vi "addTaskMethod.vi"(8 "error in":errorcluster, 10 "stopMechanismType":T1, 11 "classPath":path) -> (0 "error out":errorcluster, 2 "taskViPath":path, 3 "classPath(dup)":path)   [LabVIEW 2023]
uses:
  stopMechanismType.ctl
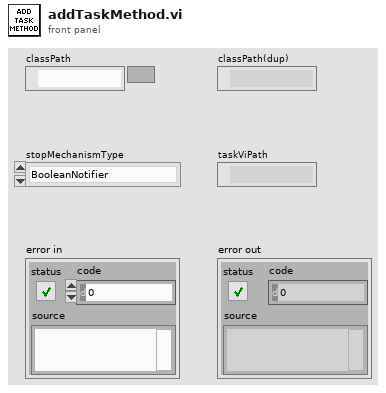
[diagram p1: front panel]
types:
  T1 = typedef "stopMechanismType.ctl" = enum16{"BooleanNotifier", "BooleanUE", "MsgUE", "MsgQueue"}
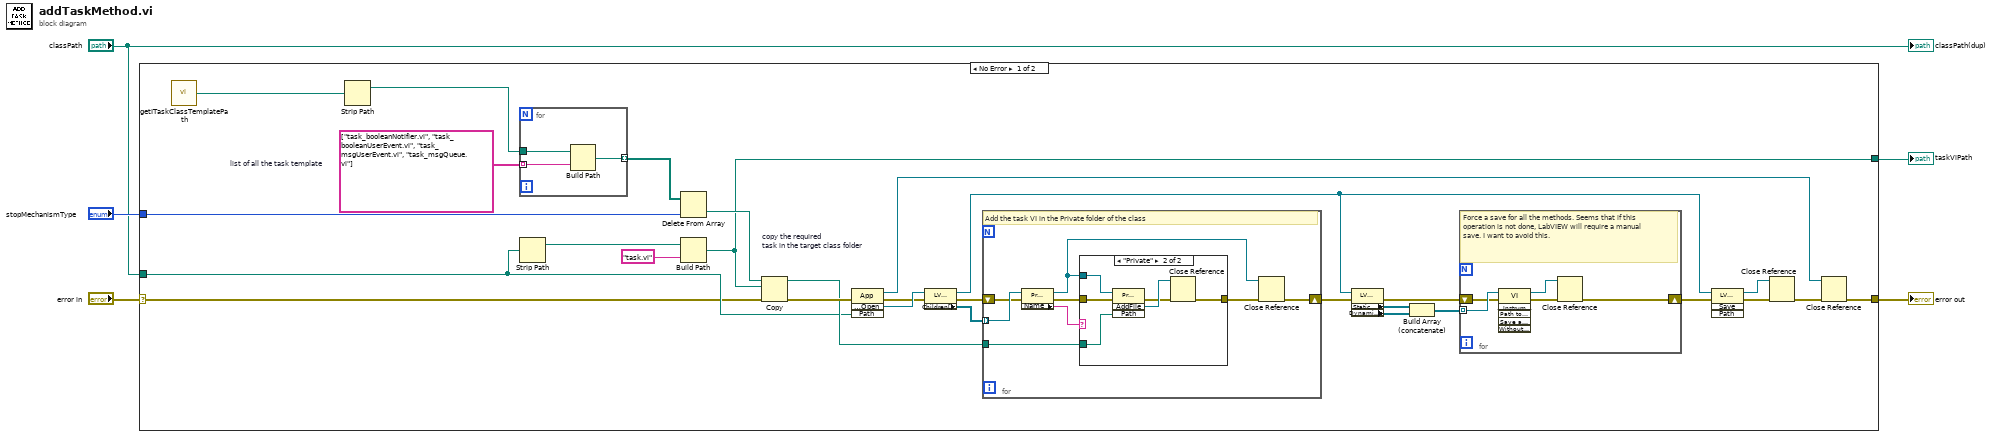
[diagram p0: block diagram]
diagram:
  n1 = case shown="No Error" "error in" {
    selector: "error in" -> [w7 w58]
    tunnel: "classPath" -> [w22 _]
    tunnel: [w20 w58] -> w5
    tunnel: "stopMechanismType" -> [w9 _]
    tunnel: [w6 _] -> w2
    frame No Error {
      w8 = string[] ["task_booleanNotifier.vi", "task_booleanUserEvent.vi", "task_msgUserEvent.vi", "task_msgQueue.vi"]  # list of all the task template
      n2 = call "getITaskClassTemplatePath.vi"() -> ("ITaskClassPath"=w10:path)
      n3 = Strip Path(path=w10) -> (stripped path=w11:path)  [unwired: 1 out]
      n4 = for {
        tunnel: w11 -> [w57]
        tunnel: w8 -> [w56] mode=indexing
        tunnel: [w55] -> w12 mode=indexing
        n5 = Build Path(base path=w57, name or relative path=w56) -> (appended path=w55:path)
      }
      n6 = Strip Path(path=w22) -> (stripped path=w23:path)  [unwired: 1 out]
      n7 = Delete From Array(array=w12, index=w9) -> (deleted portion=w25:path)  [unwired: 1 in, 1 out]
      n8 = Build Path(base path=w23, name or relative path="task.vi" ("String")) -> (appended path=w6:path)
      n9 = Copy "copy the required\ntask in the target class folder"(8:w7, 10:w6, 11:w25) -> (0:w27:errorcluster, 3:w26:path)  [unwired: 2 in, 1 out]
      n10 = invoke class="App" method="LVClass.Open"(error in=w27, "Path"=w22) -> (reference out=w21:refnum<vi>, error out=w16:errorcluster, "LVClass.Open"=w18:refnum<vi>)  [unwired: 2 in, 1 out]
      n11 = property class="LVClassLibrary"(reference=w18, error in=w16) -> (reference out=w29:refnum<vi>, error out=w17:errorcluster, "Children[]"=w13:refnum<vi>[])
      n12 = for {
        tunnel: w26 -> [w47]
        tunnel: w13 -> [w46] mode=indexing
        shift-right: [w41] -> w28
        shift-left: w17 -> [w40]
        # "Add the task VI in the Private folder of the class"
        n13 = property class="ProjectItem"(reference=w46, error in=w40) -> (reference out=w44:refnum<vi>, error out=w42:errorcluster, "Name"=w45:string)
        n14 = case shown="\"Private\"" w45 {
          tunnel: w47 -> [_ w54]
          tunnel: w44 -> [_ w53]
          tunnel: [w48 w50] -> w43
          tunnel: w42 -> [w48 w49]
          frame Default {
          }
          frame "Private" {
            n15 = invoke class="ProjectItem" method="AddFile"(reference=w53, error in=w49, "Path"=w54) -> (error out=w51:errorcluster, "AddFile"=w52:refnum<vi>)  [unwired: 1 in, 2 out]
            n16 = Close Reference(reference=w52, error in (no error)=w51) -> (error out=w50:errorcluster)
          }
        }
        n17 = Close Reference(reference=w44, error in (no error)=w43) -> (error out=w41:errorcluster)
      }
      n18 = property class="LVClassLibrary"(reference=w29, error in=w28) -> (error out=w33:errorcluster, "Static Member VIs"=w31:refnum<vi>[], "Dynamic Member VIs"=w30:refnum<vi>[])  [unwired: 1 out]
      n19 = Build Array (concatenate)(w31, w30) -> (w32:refnum<vi>[])
      n20 = for {
        tunnel: w32 -> [w39] mode=indexing
        shift-right: [w36] -> w34
        shift-left: w33 -> [w38]
        # "Force a save for all the methods. Seems that if this operation is not done, LabVIEW will require a manual save. I want to avoid this."
        n21 = invoke class="VI" method="Save.Instrument"(reference=w39, error in=w38) -> (reference out=w35:refnum<vi>, error out=w37:errorcluster)  [unwired: 4 in, 4 out]
        n22 = Close Reference(reference=w35, error in (no error)=w37) -> (error out=w36:errorcluster)
      }
      n23 = invoke class="LVClassLibrary" method="Save"(reference=w29, error in=w34) -> (reference out=w15:refnum<vi>, error out=w14:errorcluster)  [unwired: 2 in, 2 out]
      n24 = Close Reference(reference=w15, error in (no error)=w14) -> (error out=w19:errorcluster)
      n25 = Close Reference(reference=w21, error in (no error)=w19) -> (error out=w20:errorcluster)
    }
    frame Error {
    }
  }
  "error out" <- w5
  "taskViPath" <- w2
  "classPath(dup)" <- "classPath"
